vi "Calc LRC-8.vi"(3 "Frame in":u8[](array[numeric]) format="%.0x") -> (1 "LRC-8":u8 format="%.0x")   [LabVIEW 2016, in "MB Master.lvlib" / "MB_ADU_ASCII.lvclass"]
doc: "Calculates the 8-bit LRC of a Modbus ASCII ADU (<Address><Function Code><[Data]>)"
uses:
  MB_ADU_ASCII.lvclass
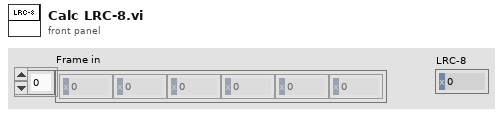
[diagram p1: front panel]
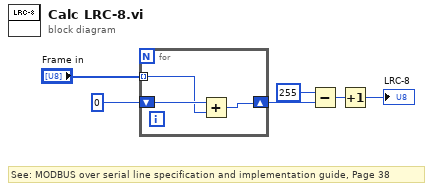
[diagram p0: block diagram]
diagram:
  # "See: MODBUS over serial line specification and implementation guide, Page 38"
  n1 = for {
    tunnel: "Frame in" -> [w8] mode=indexing
    shift-right: [w7] -> w4
    shift-left: u8 0 -> [w9]
    n2 = Add(x=w9, y=w8) -> (x+y=w7:u8)
  }
  n3 = Subtract(x=u8 255, y=w4) -> (x-y=w3:u8)
  n4 = Increment(x=w3) -> (x+1=→"LRC-8":u8)
